vi "Shift I32 Number to get block exponent number.vi"(8 "Input Valid":bool=TRUE, 10 "Leading Zero Position":u8, 11 "Binary Number":i32 format="%.0b") -> (0 "Output Valid":bool=TRUE, 2 "Block Float Exponent":i8, 3 "Block Float Mantissa":i32)   [LabVIEW 2010]
uses:
  <vilib>/rvi/FXPMathLib/basic elements/FxpDiscreteDelay/XNode/nifxpmath_DiscreteDelay.xnode
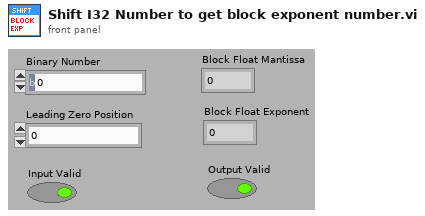
[diagram p1: front panel]
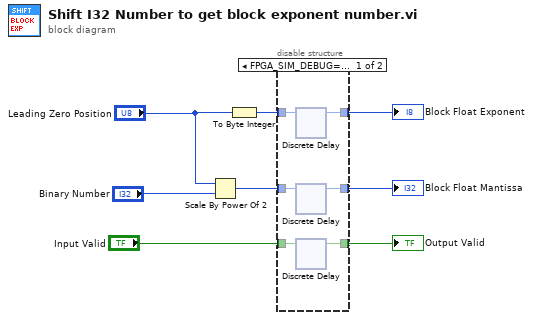
[diagram p0: block diagram]
diagram:
  n1 = Scale By Power Of 2(n="Leading Zero Position", x="Binary Number") -> (x*2^n=w6:i32)
  n2 = To Byte Integer(number="Leading Zero Position") -> (8bit integer=w5:i8)
  n3 = disable-structure shown="FPGA_SIM_DEBUG==FALSE, default" {
    disable-tunnel: w6 -> [w14 w112]
    disable-tunnel: w5 -> [w13 w113]
    disable-tunnel: "Input Valid" -> [w12 w111]
    disable-tunnel: [w11 w113] -> w3
    disable-tunnel: [w10 w112] -> w2
    disable-tunnel: [w9 w111] -> w1
    frame condition #0 {
      n4 = xnode "Discrete Delay"("D"=w13) -> ("Q"=w11:i8)
      n5 = xnode "Discrete Delay"("D"=w14) -> ("Q"=w10:i32)
      n6 = xnode "Discrete Delay"("D"=w12) -> ("Q"=w9:bool)
    }
    frame condition #1 (active) {
    }
  }
  "Block Float Mantissa" <- w2
  "Block Float Exponent" <- w3
  "Output Valid" <- w1
